vi "Get Socket Counter Name.vi"(8 "error In":errorcluster, 10 "ChannelType":string, 11 "Physical Channel":tag[](array[tag])) -> (0 "error out":errorcluster, 2 "ReferenceClock":tag[](array[tag]), 3 "CounterName":tag[](array[tag]))   [LabVIEW 2023, in "HardwareAbstractionLayer_LVOOP.lvlib" / "Teststand.lvclass"]
doc: "This VI Filter Physical Channel and Number Socket Running"
uses:
  Teststand.lvclass
  Database/Database.lvclass
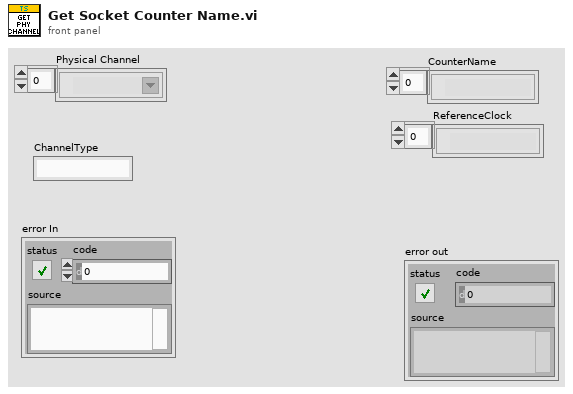
[diagram p1: front panel]
types:
  T1 = cluster{"table":string, "condition":string, "columns":string[]}
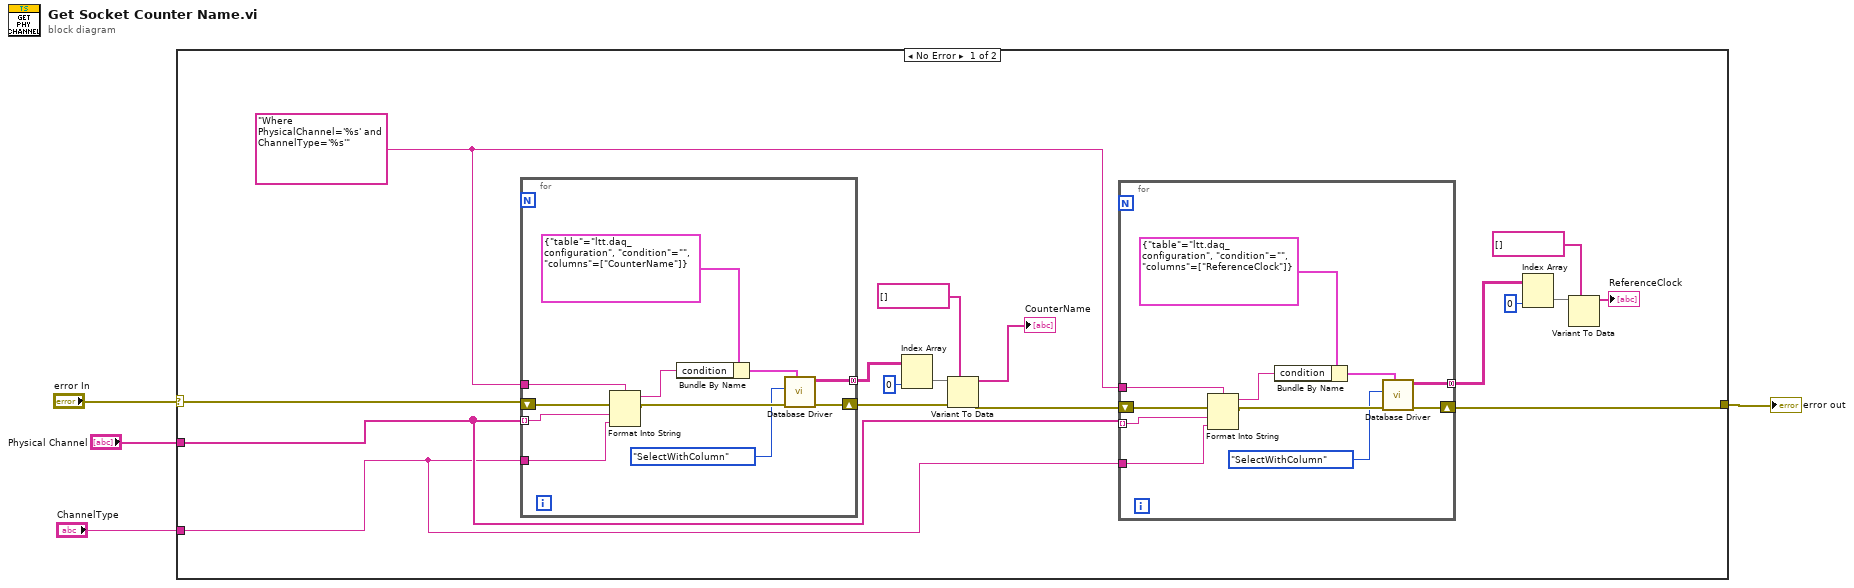
[diagram p0: block diagram]
diagram:
  n1 = case shown="No Error" "error In" {
    selector: "error In" -> [w17 w44]
    tunnel: "ChannelType" -> [w11 _]
    tunnel: [w13 w44] -> w3
    tunnel: "Physical Channel" -> [w12 _]
    frame No Error {
      w10 = "Where PhysicalChannel='%s' and ChannelType='%s'"
      n2 = for {
        tunnel: w10 -> [w43]
        shift-right: [w36] -> w21
        shift-left: w17 -> [w40]
        tunnel: [w35] -> w20 mode=concatenating
        tunnel: w11 -> [w39]
        tunnel: w12 -> [w33] mode=indexing
        n3 = Format Into String(format string=w43, error in=w40, w33, w39) -> (resulting string=w41:string, error out=w37:errorcluster)  [unwired: 1 in]
        n4 = Bundle By Name(cluster=T1 {"table"="ltt.daq_configuration", "condition"="", "columns"=["CounterName"]} ("SQLTableData"), "condition"=w41) -> (w38:T1)
        n5 = call "Database Driver.vi"("SQLTableData"=w38, "error in"=w37, "Select"=enum16{"SelectWithQuery", "SelectWithColumn"}."SelectWithColumn") -> ("error out"=w36:errorcluster, "data"=w35:string[][])  [unwired: 5 in, 2 out]
      }
      n6 = Index Array(array=w20, index (col)=0 ("disabled index (col)")) -> (element=w19:string[])  [unwired: 1 in]
      n7 = Variant To Data(error in=w21, type=tag[] [] ("AI.PhysicalChans"), Variant=w19) -> (data=→"CounterName":tag[], error out=w14:errorcluster)
      n8 = for {
        tunnel: w10 -> [w32]
        shift-right: [w25] -> w13
        shift-left: w14 -> [w29]
        tunnel: [w24] -> w7 mode=concatenating
        tunnel: w11 -> [w28]
        tunnel: w12 -> [w22] mode=indexing
        n9 = Format Into String(format string=w32, error in=w29, w22, w28) -> (resulting string=w30:string, error out=w26:errorcluster)  [unwired: 1 in]
        n10 = Bundle By Name(cluster=T1 {"table"="ltt.daq_configuration", "condition"="", "columns"=["ReferenceClock"]} ("SQLTableData"), "condition"=w30) -> (w27:T1)
        n11 = call "Database Driver.vi"("SQLTableData"=w27, "error in"=w26, "Select"=enum16{"SelectWithQuery", "SelectWithColumn"}."SelectWithColumn") -> ("error out"=w25:errorcluster, "data"=w24:string[][])  [unwired: 5 in, 2 out]
      }
      n12 = Index Array(array=w7, index (col)=0 ("disabled index (col)")) -> (element=w8:string[])  [unwired: 1 in]
      n13 = Variant To Data(type=tag[] [] ("Ref Clock"), Variant=w8) -> (data=→"ReferenceClock":tag[])  [unwired: 1 in, 1 out]
    }
    frame Error {
    }
  }
  "error out" <- w3
